vi "Update Type in Tree.vi"(6 "Type":T1, 8 "error in (no error)":errorcluster, 9 "DC_UID":T2, 10 "WID":string, 11 "Tree Ref":refnum<vi>) -> (0 "error out":errorcluster)   [LabVIEW 2017, in "Application Manager.lvclass"]
uses:
  Application Manager.lvclass
  Common VIs/DC_UID.ctl
  <vilib>/addons/_Workers/Library/Classes/Worker/Worker Type.ctl
  <vilib>/addons/_Workers/Library/Classes/Worker/Worker.lvclass
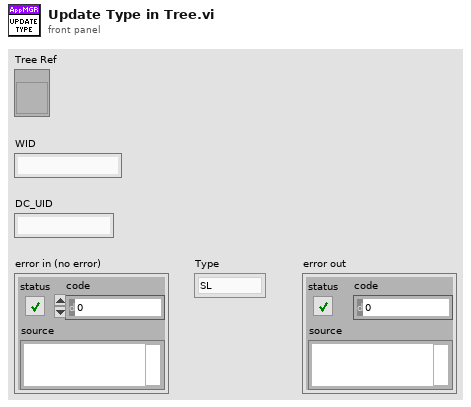
[diagram p1: front panel]
types:
  T1 = typedef "Workers.lvlib/Worker.lvclass/Worker Type.ctl" = enum16{"SL", "DL"}
  T2 = typedef "DC_UID.ctl" = string
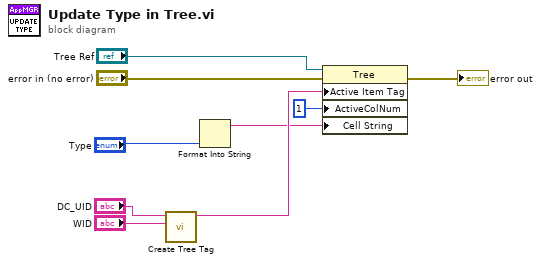
[diagram p0: block diagram]
diagram:
  n1 = call "Create Tree Tag.vi"("WID"="WID", "DC_UID"="DC_UID") -> ("Tree Tag"=w3:string)  [unwired: 9 in]
  n2 = Format Into String("Type") -> (resulting string=w1:string)  [unwired: 3 in, 1 out]
  n3 = property class="Tree"(reference="Tree Ref", error in="error in (no error)", "Active Item Tag"=w3, "ActiveColNum"=1 ("Active Cell:Active Column Number"), "Cell String"=w1) -> (error out=→"error out":errorcluster)  [unwired: 1 out]
